vi "Log String Message.vi"(8 "Error In":errorcluster, 10 "Message":string, 11 "FileLogger In":refnum<class "FileLogger.lvclass">) -> (0 "Error Out":errorcluster, 3 "FileLogger Out":refnum<class "FileLogger.lvclass">)   [LabVIEW 2019, in "FileLogger.lvclass"]
uses:
  FileLogger.lvclass
  FileLogger.lvclass/FileLogger.ctl
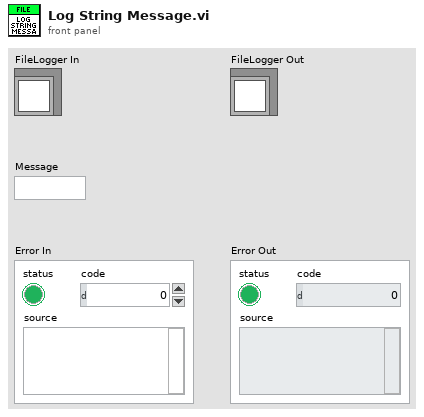
[diagram p1: front panel]
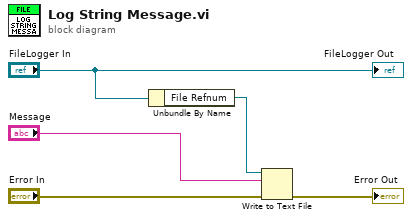
[diagram p0: block diagram]
diagram:
  n1 = Unbundle By Name("FileLogger In") -> ("File Refnum"=w4:refnum<file>)
  n2 = Write to Text File(file (use dialog)=w4, text="Message", error in="Error In") -> (error out=→"Error Out":errorcluster)  [unwired: 1 in, 2 out]
  "FileLogger Out" <- "FileLogger In"
